vi "Global_vars.vi"() -> ()   [LabVIEW 2019]
panel:
  out "counter_seq":dbl
  out "Nerve_block":bool
  out "NerveBlock":dbl
  in  "Sin Sq":bool
  out "Band":dbl
  out "KI":dbl
  out "KP":dbl
  in  "Fuzzy_comp":dbl
  out "yk":dbl
  in  "maxCS":dbl
  in  "minCS":dbl
  in  "Ref offset":dbl
  in  "Ref amp":dbl
  out "Gff save":dbl
  in  "model onoff save":bool
  out "control signal fb":dbl
  out "control signal ff":dbl
  in  "F trans":dbl[](array[numeric])
  out "PW":dbl[](array[numeric])
  out "stim freq save":dbl
  out "offset save":dbl
  out "ref amp save":dbl
  out "ref freq save":dbl
  out "amplitude save":dbl
  in  "PID gains save":T1={"proportional gain (Kc)"=1.0, "integral time (Ti, min)"=0.01, "derivative time (Td, min)"=0.0} {"derivative time (Td, min)" format="%.3f"; "integral time (Ti, min)" format="%.3f"; "proportional gain (Kc)" format="%.3f"}
  in  "Mode test CL":bool
  out "control variable":dbl
  out "control signal":dbl
  out "raw F":dbl
  in  "stop":bool
  out "F ref":dbl
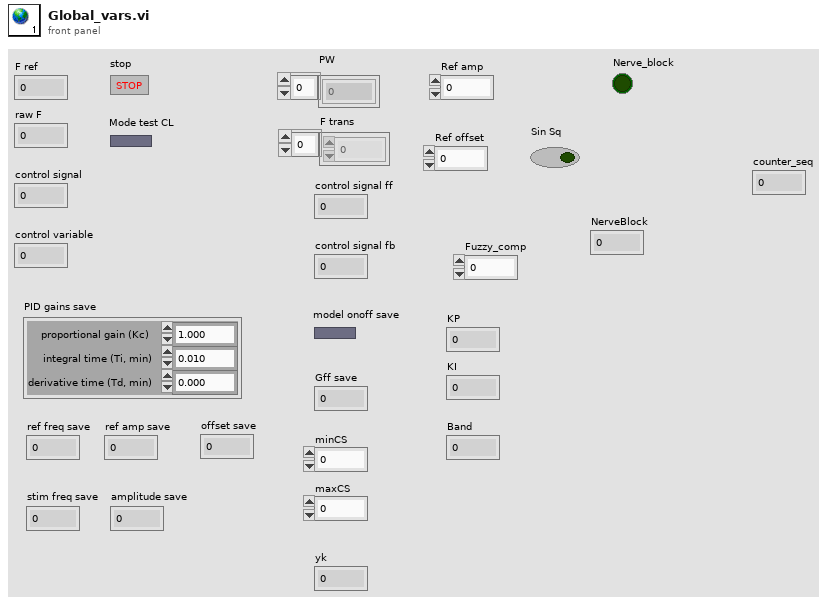
[diagram p1: front panel]
types:
  T1 = cluster{"proportional gain (Kc)":dbl, "integral time (Ti, min)":dbl, "derivative time (Td, min)":dbl}
diagram:
